vi "MV warm-up.vi"(8 "error in (no error)":errorcluster, 10 "slide indicator reference":refnum<vi>, 11 "VISA resource name":refnum<visa-resource-name>) -> (0 "error out":errorcluster, 3 "VISA resource name out":refnum<visa-resource-name>)   [LabVIEW 2015, in "Millennia V.lvclass"]
doc: "Warms up the Millennia V laser and then terminates once it's fully warmed up. You can optionally wire in a reference to a slide indicator which will be updated continuously with the current status of the laser."
uses:
  Millennia V.lvclass
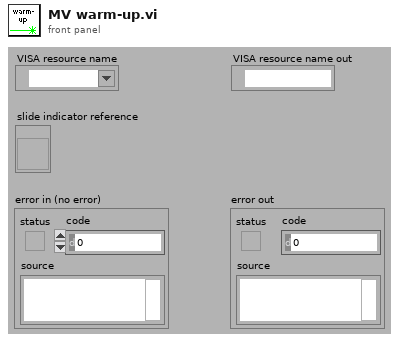
[diagram p1: front panel]
types:
  T1 = enum16{"read only", "write only", "write + read"}
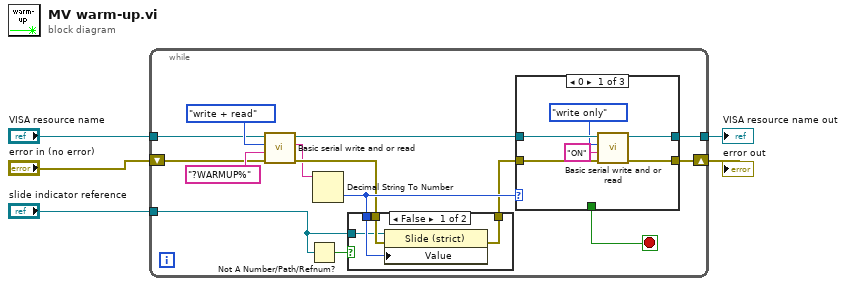
[diagram p0: block diagram]
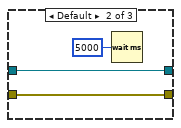
[diagram p3: hidden frame]
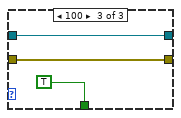
[diagram p4: hidden frame]
diagram:
  n1 = while {
    tunnel: "VISA resource name" -> [w16]
    shift-right: [w13] -> w2
    shift-left: "error in (no error)" -> [w15]
    tunnel: [w14] -> w3
    tunnel: "slide indicator reference" -> [w8]
    stop <- w12 stop-if-true
    n2 = call "Basic serial write and or read.vi"("error in (no error)"=w15, "write string"="?WARMUP%", "action"=T1."write + read", "VISA resource name"=w16) -> ("error out"=w10:errorcluster, "read string"=w6:string, "VISA resource name out"=w17:refnum<visa-resource-name>)  [unwired: 4 in, 1 out]
    n3 = Not A Number/Path/Refnum?(number/path/refnum=w8) -> (NaN/Path/Refnum?=w7:bool)
    n4 = Decimal String To Number(string=w6) -> (number=w11:i32)  [unwired: 2 in, 1 out]
    n5 = case shown="False" w7 {
      tunnel: w11 -> [w23 _]
      tunnel: w10 -> [w22 w24]
      tunnel: [w21 w24] -> w9
      tunnel: w8 -> [w20 _]
      frame False {
        n6 = property class="Slide (strict)"(reference=w20, error in=w22, "Value"=w23) -> (error out=w21:errorcluster)  [unwired: 1 out]
      }
      frame True {
      }
    }
    n7 = case shown="0" w11 {
      tunnel: w9 -> [w29 w31 w34]
      tunnel: w17 -> [w30 w32 w35]
      tunnel: [w26 w32 w35] -> w14
      tunnel: [w25 w31 w34] -> w13
      tunnel: [_ _ TRUE] -> w12
      frame 0 {
        n8 = call "Basic serial write and or read.vi"("error in (no error)"=w29, "write string"="ON", "action"=T1."write only", "VISA resource name"=w30) -> ("error out"=w25:errorcluster, "VISA resource name out"=w26:refnum<visa-resource-name>)  [unwired: 4 in, 2 out]
      }
      frame Default {
        n9 = Wait (ms)(milliseconds to wait=u32 5000) -> ()  [unwired: 1 out]
      }
      frame 100 {
      }
    }
  }
  "VISA resource name out" <- w3
  "error out" <- w2
